vi "模块启用设置.vi"() -> ()   [LabVIEW 2016]
uses:
  <vilib>/Utility/miscctls.llb/LVPointTypeDef.ctl
  <vilib>/Utility/config.llb/NI_LVConfig.lvlib
panel:
  in  "原位多参数":bool=TRUE
  in  "确认":bool
  in  "营养盐":bool=TRUE
  in  "集成式多参数":bool=TRUE
  # "请选择要启用的模块"
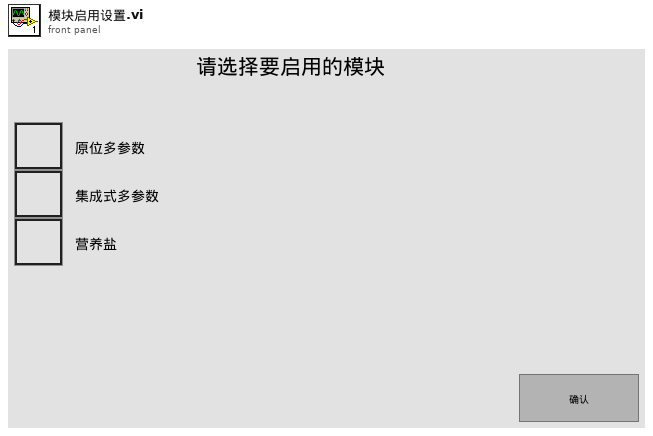
[diagram p1: front panel]
types:
  T1 = typedef "LVPointTypeDef.ctl" = cluster{"Horizontal":i16, "Vertical":i16}
  T2 = typedef "NI_LVConfig.lvlib/Config Data RefNum.ctl" = refnum<k1>
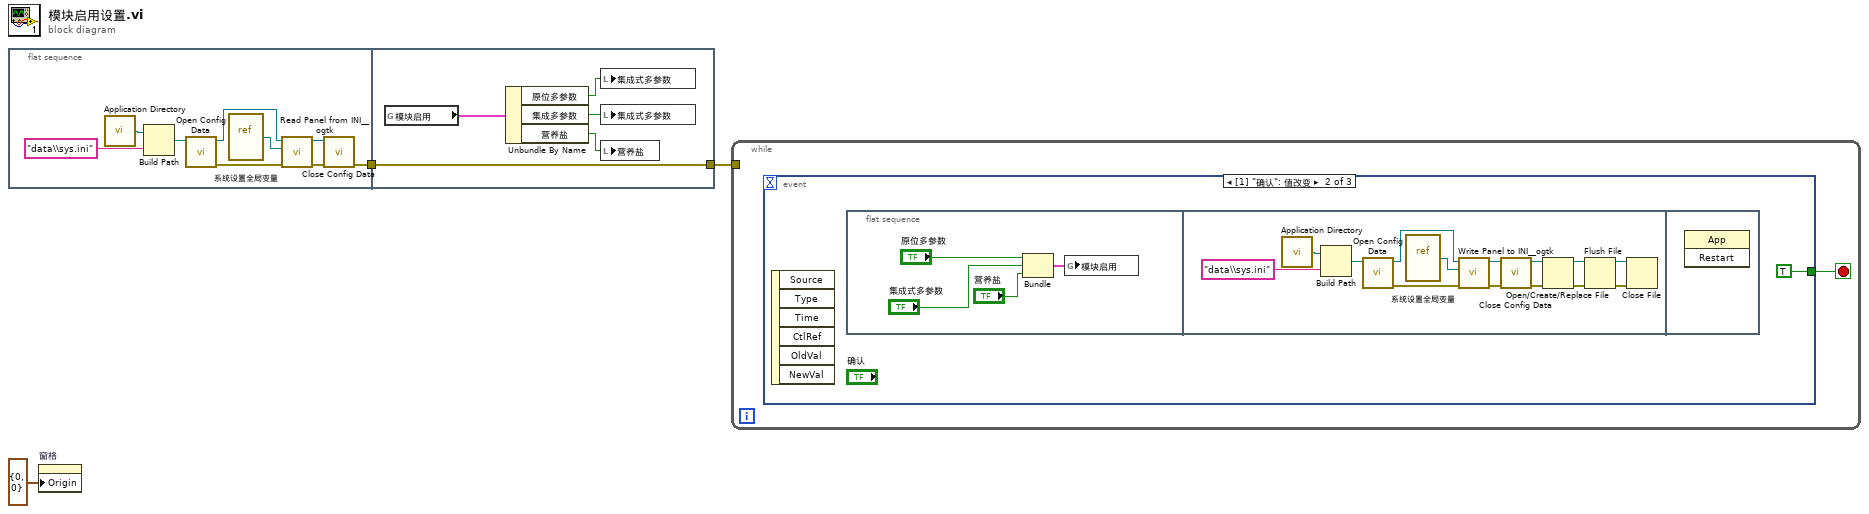
[diagram p0: block diagram]
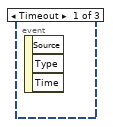
[diagram p2: hidden frame]
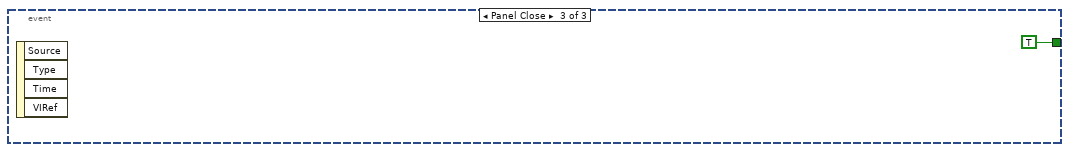
[diagram p3: hidden frame]
diagram:
  n1 = flat-sequence {
    tunnel: [w4] -> w2
    tunnel: w2 -> [w17]
    tunnel: [w17] -> w1
    frame #0 {
      n2 = call <vilib>:"Application Directory.vi"() -> ("Application Directory"=w12:path)
      n3 = Build Path(base path=w12, name or relative path="data\\sys.ini" ("名称或相对路径")) -> (appended path=w10:path)
      n4 = call <vilib>:"Open Config Data.vi"("configuration file path"=w10) -> ("error out"=w6:errorcluster, "refnum"=w9:T2)  [unwired: 8 in, 1 out]
      n5 = vi-ref "系统设置全局变量.vi"() -> (w8:refnum<vi>)
      n6 = call <userlib>:"Read Panel from INI__ogtk.vi"("error in (no error)"=w6, "VI ref"=w8, "refnum"=w9) -> ("error out"=w5:errorcluster, "refnum out"=w7:T2)  [unwired: 7 in]
      n7 = call <vilib>:"Close Config Data.vi"("error in (no error)"=w5, "refnum"=w7) -> ("error out"=w4:errorcluster)  [unwired: 8 in, 1 out]
    }
    frame #1 {
      n8 = global read "系统设置全局变量.vi" "模块启用"() -> (w16:cluster{"原位多参数":bool, "集成多参数":bool, "营养盐":bool})
      n9 = Unbundle By Name(w16) -> ("原位多参数"=w15:bool, "集成多参数"=w14:bool, "营养盐"=w13:bool)
      n10 = local write "集成式多参数"(w15) -> ()
      n11 = local write "集成式多参数"(w14) -> ()
      n12 = local write "营养盐"(w13) -> ()
    }
  }
  n13 = property on="窗格" class="Pane"("Origin"=T1 {"Horizontal"=0, "Vertical"=0} ("原点")) -> ()  [unwired: 2 in, 2 out]
  n14 = while {
    tunnel: w1 -> [_]
    stop <- w18 stop-if-true
    n15 = event shown="[1] \"确认\": 值改变" {
      selector: _ -> [_ _ _]
      dyn-events: _ -> [_ _ _]
      timeout: _ -> [_ _ _]
      tunnel: [_ TRUE TRUE] -> w18
      event Timeout {
        n16 = event-data() -> ()  [unwired: 1 in, 3 out]
      }
      event "确认": Value Change {
        n17 = event-data() -> ()  [unwired: 1 in, 6 out]
        n18 = flat-sequence {
          frame #0 {
            n19 = Bundle("原位多参数"="原位多参数", "集成式多参数"="集成式多参数", "营养盐"="营养盐") -> (w20:cluster{"原位多参数":bool, "集成式多参数":bool, "营养盐":bool})  [unwired: 1 in]
            n20 = global write "系统设置全局变量.vi" "模块启用"(w20) -> ()
          }
          frame #1 {
            n21 = call <vilib>:"Application Directory.vi"() -> ("Application Directory"=w24:path)
            n22 = Build Path(base path=w24, name or relative path="data\\sys.ini" ("名称或相对路径")) -> (appended path=w26:path)
            n23 = call <vilib>:"Open Config Data.vi"("configuration file path"=w26) -> ("error out"=w30:errorcluster, "refnum"=w27:T2)  [unwired: 8 in, 1 out]
            n24 = vi-ref "系统设置全局变量.vi"() -> (w28:refnum<vi>)
            n25 = call <userlib>:"Write Panel to INI__ogtk.vi"("error in (no error)"=w30, "VI ref"=w28, "refnum"=w27) -> ("error out"=w31:errorcluster, "refnum out"=w29:T2)  [unwired: 7 in]
            n26 = call <vilib>:"Close Config Data.vi"("error in (no error)"=w31, "refnum"=w29) -> ("error out"=w36:errorcluster, "file path"=w37:path)  [unwired: 8 in]
            n27 = Open/Create/Replace File(file path (use dialog)=w37, error in=w36) -> (refnum out=w33:refnum<file>, error out=w32:errorcluster)  [unwired: 4 in, 1 out]
            n28 = Flush File(refnum=w33, error in=w32) -> (refnum out=w34:refnum<file>, error out=w35:errorcluster)
            n29 = Close File(refnum=w34, error in=w35) -> ()  [unwired: 2 out]
          }
          frame #2 {
            n30 = invoke class="App" method="Restart"() -> ()  [unwired: 3 in, 3 out]
          }
        }
      }
      event Panel Close {
        n31 = event-data() -> ()  [unwired: 1 in, 4 out]
      }
    }
  }
